vi "RectWindow.vi"(8 "error in":errorcluster, 11 "np":dbl=256.0) -> (0 "error out":errorcluster, 3 "win":dbl[](graph))   [LabVIEW 2009]
uses:
  <vilib>/imath/engines/lvmath2/RunTimeEngine/ErrorHandling/NIMS_Finalize Error.vi
  <vilib>/imath/engines/lvmath2/RunTimeEngine/Parser/MC_Version.vi
  <vilib>/imath/engines/lvmath2/RunTimeEngine/NodeEndStatement/NIMS_NodeEndStatement_Output.vi
  <instcachedir>/0/NIMS_NodeEndStatement_Output_53EC0D466D134D7ABD903AC30B43404B.lvgen/NIMS_NodeEndStatement_Output_53EC0D466D134D7ABD903AC30B43404B_001.vi
  <vilib>/imath/engines/lvmath2/RunTimeEngine/NodeEndStatement/NIMS_NodeEndStatement_Get Vector.vi
  <instcachedir>/0/NIMS_NodeEndStatement_Get Vector_708AE642CFEE4B9892E482CBBBA3A4D6.lvgen/NIMS_NodeEndStatement_Get Vector_708AE642CFEE4B9892E482CBBBA3A4D6_001.vi
  <vilib>/imath/engines/lvmath/Plug In/_Char/NIMS_CH_character datatype.ctl
  <vilib>/imath/engines/lvmath/Functions/Error Handling/MergeErrorsWrapper.vi
  <vilib>/imathl/engines/lvmath/Functions/Error Handling/Create Error.vi
  <vilib>/imath/engines/lvmath2/RunTimeEngine/BuiltInFunctions/random/NIMS_random.vi
  <vilib>/imath/engines/lvmath/Plug In/_Char/NIMS_CH_Character RV to String.vi
  <vilib>/imath/engines/lvmath2/RunTimeEngine/RangeToken/NIMS_Range_R2 - Float.vi
  <instcachedir>/0/NIMS_Range_R2 - Float_93A1434467634702BCAD427B3499A8B4.lvgen/NIMS_Range_R2 - Float_93A1434467634702BCAD427B3499A8B4_000.vi
  <vilib>/imath/engines/lvmath2/RunTimeEngine/ReplaceToken/NIMS_Replace - V(S)=S.vi
  <instcachedir>/0/NIMS_Replace - V(S)=S_1F711D65782C407D901BB57589CB2660.lvgen/NIMS_Replace - V(S)=S_1F711D65782C407D901BB57589CB2660_002.vi
  <vilib>/imath/engines/lvmath2/RunTimeEngine/ReplaceToken/NIMS_Replace - Size Check _(_)=S.vi
  <instcachedir>/0/NIMS_Replace - Size Check _(_)=S_C93E24300E2D4FA1B1057E3B3E42F8F7.lvgen/NIMS_Replace - Size Check _(_)=S_C93E24300E2D4FA1B1057E3B3E42F8F7_004.vi
  <vilib>/imath/engines/lvmath2/RunTimeEngine/ReplaceToken/NIMS_Replace - Check(_) Linear.vi
  <instcachedir>/0/NIMS_Replace - Check(_) Linear_E275C9AF2D6949DA8BBA624A5DF43407.lvgen/NIMS_Replace - Check(_) Linear_E275C9AF2D6949DA8BBA624A5DF43407_005.vi
  <vilib>/imath/engines/lvmath2/RunTimeEngine/VariableToken/NIMS_VariableToken_CondDefinedDefinedByReplace.vi
  <instcachedir>/0/NIMS_VariableToken_CondDefinedDefinedByReplace_D162CFFC24174562A9FEA619A91E1A56.lvgen/NIMS_VariableToken_CondDefinedDefinedByReplace_D162CFFC24174562A9FEA619A91E1A56_001.vi
  <vilib>/imath/engines/lvmath2/RunTimeEngine/CommandStatement/MC_CommandStatement_break.vi
  <vilib>/imath/engines/lvmath2/RunTimeEngine/ArithmeticOperatorToken/NIMS_ArithmeticOperator_plus.vi
  <instcachedir>/0/NIMS_ArithmeticOperator_plus_48B9519178ED42D7840F01273E784BFE.lvgen/NIMS_ArithmeticOperator_plus_48B9519178ED42D7840F01273E784BFE_009.vi
  <vilib>/imath/engines/lvmath2/RunTimeEngine/VariableToken/NIMS_VariableToken_CondDefined.vi
  <instcachedir>/0/NIMS_VariableToken_CondDefined_8A7BE13368864D8DBC6F49EC23B20D8F.lvgen/NIMS_VariableToken_CondDefined_8A7BE13368864D8DBC6F49EC23B20D8F_001.vi
  <vilib>/imath/engines/lvmath/Functions/Error Handling/MC_Error Cluster From Error Code.vi
  <vilib>/imath/engines/lvmath2/RunTimeEngine/BuiltInFunctions/abs/NIMS_abs(signed).vi
  <instcachedir>/0/NIMS_abs(signed)_C4FCB8E6058B49B797C7C8D53CA5F6EC.lvgen/NIMS_abs(signed)_C4FCB8E6058B49B797C7C8D53CA5F6EC_002.vi
  <vilib>/imath/engines/lvmath2/RunTimeEngine/BuiltInFunctions/fft/NIMS_fft(GM).vi
  <instcachedir>/0/NIMS_fft(GM)_D61006EB97DF48D4B7BC0A22887DF931.lvgen/NIMS_fft(GM)_D61006EB97DF48D4B7BC0A22887DF931_000.vi
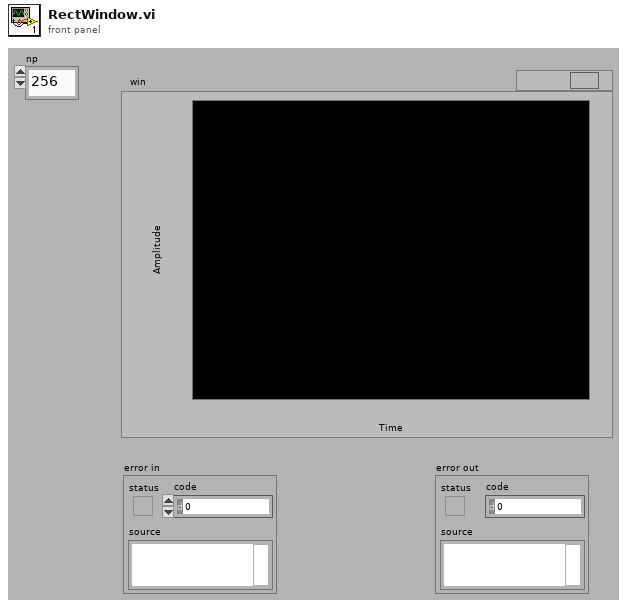
[diagram p1: front panel]
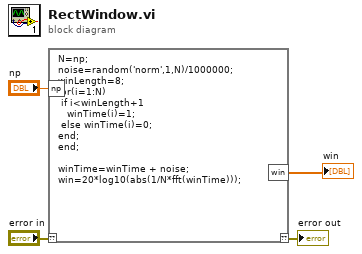
[diagram p0: block diagram]
diagram:
  n1 = mathscript code="N=np;\nnoise=random('norm',1,N)/1000000;\nwinLength=8;\nfor(i=1:N)\n if i<winLength+1\n   winTime(i)=1;\n else winTime(i)=0;\nend;\nend;\n\nwinTime=winTime + noise;\nwin=20*log10(abs(1/N*fft(winTime)));"("??"="error in", "np"="np") -> ("??"=→"error out":errorcluster, "win"=→"win":dbl[])
